vi "Write Play at Startup.vi"(10 "Play at Startup?":bool, 11 "SimpleRootModel in":refnum<class "SimpleRootModel.lvclass">) -> (3 "SimpleRootModel out":refnum<class "SimpleRootModel.lvclass">)   [LabVIEW 2017, in "MVAExamples.lvlib" / "SimpleRootModel.lvclass"]
uses:
  SimpleRootModel.lvclass
  SimpleRootModel.lvclass/SimpleRootModel.ctl
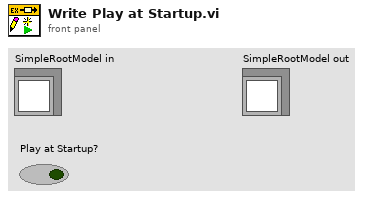
[diagram p1: front panel]
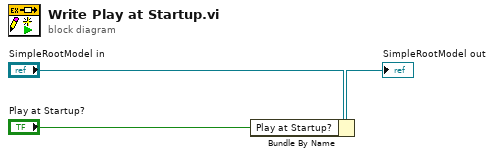
[diagram p0: block diagram]
diagram:
  n1 = Bundle By Name(cluster="SimpleRootModel in", "Play at Startup?"="Play at Startup?") -> (→"SimpleRootModel out":refnum<class "SimpleRootModel.lvclass">)
